vi "XML Scripter ValVariants Global.vi"() -> ()   [LabVIEW 2021]
panel:
  out "ValVariants []":variant[](array[variant])
  # "This global contains the ValVariants [] array\nnecessary for the XML Scripter. For each Control/\nIndicator/Constant scripted, the user must insert\na corresponsing variant containing the datatype \nand value in the designated location in the \nValVariants [] array"
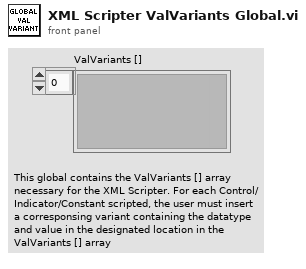
[diagram p1: front panel]
diagram:
